vi "Keithley 27XX Single Measurement.vi"() -> ()   [LabVIEW 2020]
doc: "This example VI allows you to configure a single point measurement, and returns the result of that measurement.\n\nNote:\nFor front panel measurements, make sure the Input switch is in the out position(F)\nFor plug-in card measurements, make sure the Input switch is in the in poisition(R)"
uses:
  <instrlib>/Keithley 27XX/Public/Data/Read Single Point.vi
  <instrlib>/Keithley 27XX/Keithley 27XX.lvlib
panel:
  in  "Serial Configuration":T1={"Baud Rate (9600)"=9600, "Flow Control (1: XON/XOFF)"=1, "Termination Char (0:CR)"=0} {"Termination Char (0:CR)" items=["CR", "LF"]; "Flow Control (1: XON/XOFF)" items=["None", "XON/XOFF", "RTS/CTS (2701 Only)", "XON/XOFF & RTS/CTS (2701 Only)"]; "Baud Rate (9600)" items=["300"=300, "600"=600, "1200"=1200, "2400"=2400, "4800"=4800, "9600"=9600, "19.2k"=19200, "38.4k (2701 Only)"=38400, "57.6k (2701 Only)"=57600, "115.2k (2701 Only)"=115200]}
  in  "Scan List (Empty: front panel)":string
  in  "VISA resource name":refnum<visa-resource-name>
  in  "Function (0: DC Voltage)":u16(ring) items=["DC Voltage", "AC Voltage", "DC Current", "AC Current", "Resistance", "Four-Wire Resistance", "Temperature (C)", "Frequency", "Period", "Continuity"]
  out "Measurement Data":dbl
  # "*For front panel measurements, make sure the Input switch is in the out position(F)*\n  For plug-in card measurements, make sure the Input switch is in the in position(R)"
  # "© 2005 National Instruments Corporation.  ALL RIGHTS RESERVED."
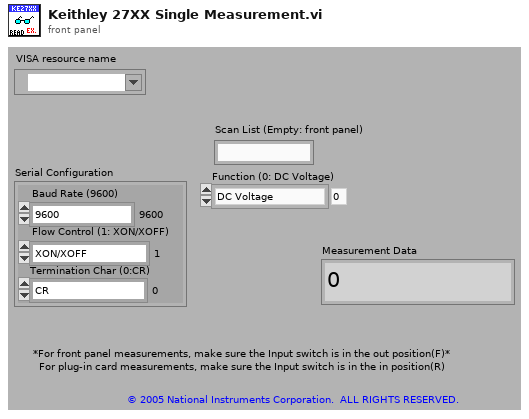
[diagram p1: front panel]
types:
  T1 = cluster{"Baud Rate (9600)":u32, "Flow Control (1: XON/XOFF)":u16, "Termination Char (0:CR)":u16}
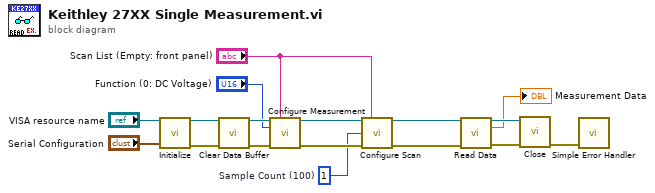
[diagram p0: block diagram]
diagram:
  w7 = 1  # Sample Count (100)
  n1 = call <instrlib>:"Initialize.vi"("VISA resource name"="VISA resource name", "Serial Configuration"="Serial Configuration") -> ("VISA resource name out"=w4:refnum<visa-resource-name>, "error out"=w3:errorcluster)  [unwired: 12 in]
  n2 = call <instrlib>:"Clear Data Buffer.vi"("VISA resource name"=w4, "error in (no error)"=w3) -> ("VISA resource name out"=w10:refnum<visa-resource-name>, "error out"=w11:errorcluster)  [unwired: 12 in]
  n3 = call <instrlib>:"Configure Measurement.vi"("VISA resource name"=w10, "Scan List (Empty)"="Scan List (Empty: front panel)", "Function (0: DC Voltage)"="Function (0: DC Voltage)", "error in (no error)"=w11) -> ("VISA resource name out"=w13:refnum<visa-resource-name>, "error out"=w12:errorcluster)  [unwired: 10 in]
  n4 = call <instrlib>:"Configure Scan.vi"("VISA resource name"=w13, "Channel List (101:110)"="Scan List (Empty: front panel)", "Sample Count (100)"=w7, "error in (no error)"=w12) -> ("VISA resource name out"=w8:refnum<visa-resource-name>, "error out"=w9:errorcluster)  [unwired: 10 in]
  n5 = call-poly <instrlib>:"Read Data.vi"("VISA resource name"=w8, "error in (no error)"=w9) -> ("VISA resource name out"=w16:refnum<visa-resource-name>, "Measurement Data"=→"Measurement Data":dbl, "error out"=w15:errorcluster)  [unwired: 11 in]
  n6 = call <instrlib>:"Close.vi"("VISA resource name"=w16, "error in (no error)"=w15) -> ("error out"=w14:errorcluster)  [unwired: 13 in]
  n7 = call <vilib>:"Simple Error Handler.vi"("error in (no error)"=w14) -> ()  [unwired: 4 in, 5 out]
